vi "Unescape_String.vi"(1 "Input String":string) -> (0 "Output String":string)   [LabVIEW 2011]
doc: "This VI will remove all escape sequences from the input string and replace them with their non-escaped counterparts. For example, an input of \"\\(Test\\)\" (without quotes) would yield an output of \"(Test)\"."
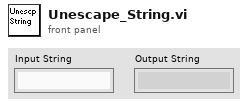
[diagram p1: front panel]
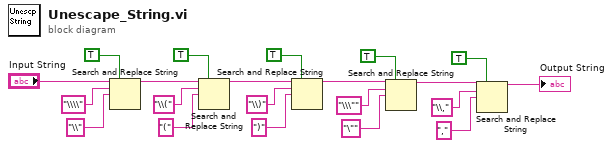
[diagram p0: block diagram]
diagram:
  n1 = Search and Replace String(replace all?=TRUE ("replace all? (F)"), input string="Input String", search string="\\\\" ("input string"), replace string="\\" ("replace string (\"\")")) -> (result string=w14:string)  [unwired: 4 in, 3 out]
  n2 = Search and Replace String(replace all?=TRUE ("replace all? (F)"), input string=w14, search string="\\(" ("input string"), replace string="(" ("replace string (\"\")")) -> (result string=w10:string)  [unwired: 4 in, 3 out]
  n3 = Search and Replace String(replace all?=TRUE ("replace all? (F)"), input string=w10, search string="\\)" ("input string"), replace string=")" ("replace string (\"\")")) -> (result string=w6:string)  [unwired: 4 in, 3 out]
  n4 = Search and Replace String(replace all?=TRUE ("replace all? (F)"), input string=w6, search string="\\\"" ("input string"), replace string="\"" ("replace string (\"\")")) -> (result string=w2:string)  [unwired: 4 in, 3 out]
  n5 = Search and Replace String(replace all?=TRUE ("replace all? (F)"), input string=w2, search string="\\," ("input string"), replace string="," ("replace string (\"\")")) -> (result string=→"Output String":string)  [unwired: 4 in, 3 out]
